vi "report results.vi"(8 "error in":errorcluster, 10 "result":refnum<class "result.lvclass">, 11 "close reference and report in":refnum<class "close reference and report.lvclass">) -> (0 "error out":errorcluster, 3 "close reference and report out":refnum<class "close reference and report.lvclass">)   [LabVIEW 2013, in "close reference and report.lvclass"]
uses:
  close reference and report.lvclass
  result/result.lvclass
  close reference and report.lvclass/close reference and report.ctl
  results reporter/results reporter.lvclass
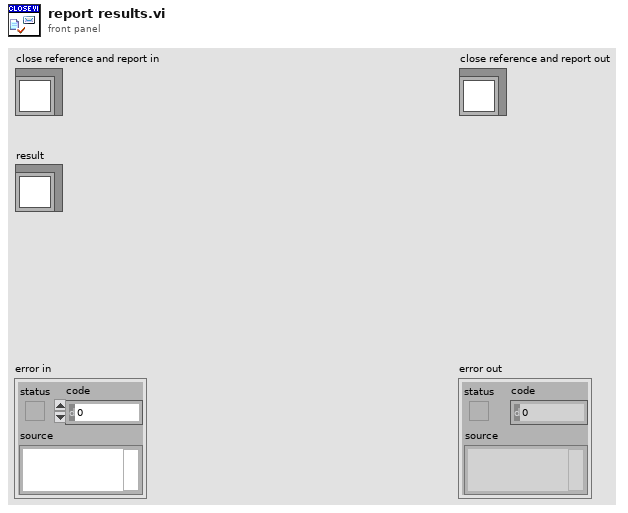
[diagram p1: front panel]
types:
  T1 = typedef "call by reference action.lvclass/function definition.ctl" = refnum<vi>
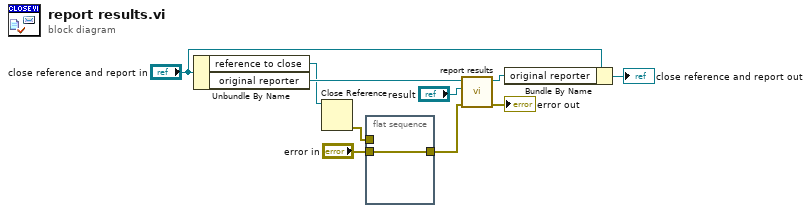
[diagram p0: block diagram]
diagram:
  n1 = Unbundle By Name("close reference and report in") -> ("reference to close"=w4:T1, "original reporter"=w8:refnum<class "results reporter.lvclass">)
  n2 = Close Reference(reference=w4) -> (error out=w3:errorcluster)  [unwired: 1 in]
  n3 = flat-sequence {
    tunnel: w3 -> [_]
    tunnel: [w11] -> w2
    tunnel: "error in" -> [w11]
    frame #0 {
    }
  }
  n4 = call-dynamic "report results.vi"("error in"=w2, "result"="result", "results reporter in"=w8) -> ("error out"=→"error out":errorcluster, "results reporter out"=w6:refnum<class "results reporter.lvclass">)  [unwired: 7 in]
  n5 = Bundle By Name(cluster="close reference and report in", "original reporter"=w6) -> (→"close reference and report out":refnum<class "close reference and report.lvclass">)
